vi "Display Module Info.vi"(8 "error IO":errorcluster, 11 "Array":refnum<class "Module.lvclass">[](array[class])) -> (0 "error out":errorcluster, 3 "Array 2":refnum<class "Module.lvclass">[](array[class]))   [LabVIEW 2021, in "Module.lvclass"]
uses:
  Module.lvclass
  Module.lvclass/Module.ctl
  <vilib>/printing/OpenHTMLReport.llb/Open HTML Report in Browser (Refnum).vi
  <vilib>/Utility/NIReport.llb/NI_report.lvclass
  <vilib>/Utility/NIReport.llb/NI_ReportGenerationCore.lvlib
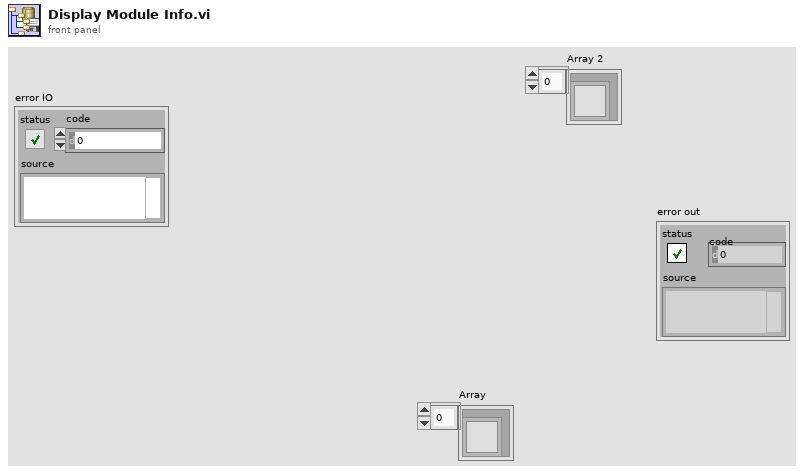
[diagram p1: front panel]
types:
  T1 = enum16{"Standard Report", "HTML", "Word", "Excel"}
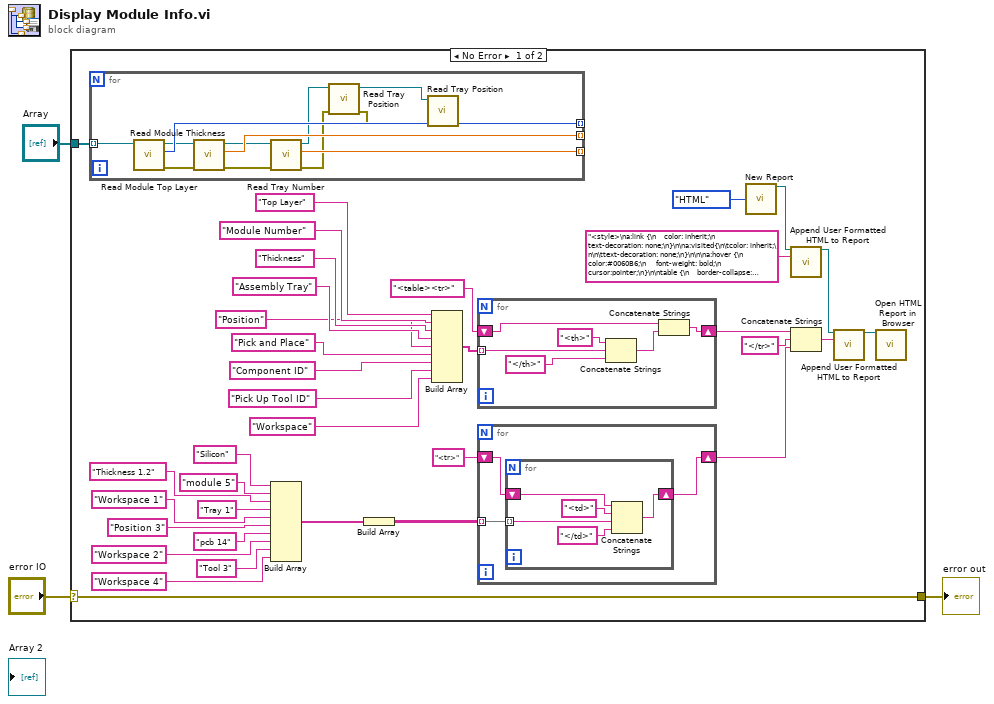
[diagram p0: block diagram]
diagram:
  n1 = case shown="No Error" "error IO" {
    selector: "error IO" -> [w38 w65]
    tunnel: [w38 w65] -> w3
    tunnel: "Array" -> [w4 _]
    frame No Error {
      n2 = for {
        tunnel: w4 -> [w50] mode=indexing
        tunnel: [w49] -> _ mode=indexing
        tunnel: [w46] -> _ mode=indexing
        tunnel: [w43] -> _ mode=indexing
        n3 = call "Read Module Top Layer.vi"("Module in"=w50) -> ("error out"=w48:errorcluster, "Module Top Layer"=w49:enum16{"Baseplate", "Kapton", "Sensor", "PCB"}, "Module out"=w47:refnum<class "Module.lvclass">)  [unwired: 8 in]
        n4 = call "Read Module Thickness.vi"("error in (no error)"=w48, "Module in"=w47) -> ("error out"=w44:errorcluster, "Module Thickness"=w46:dbl, "Module out"=w45:refnum<class "Module.lvclass">)  [unwired: 7 in]
        n5 = call "Read Tray Number.vi"("error in (no error)"=w44, "Module in"=w45) -> ("error out"=w41:errorcluster, "Tray Number"=w43:dbl, "Module out"=w42:refnum<class "Module.lvclass">)  [unwired: 7 in]
        n6 = call "Read Tray Position.vi"("error in (no error)"=w41, "Module in"=w42) -> ("error out"=w39:errorcluster, "Module out"=w40:refnum<class "Module.lvclass">)  [unwired: 7 in, 1 out]
        n7 = call "Read Tray Position.vi"("error in (no error)"=w39, "Module in"=w40) -> ()  [unwired: 7 in, 3 out]
      }
      n8 = Build Array("Silicon" ("element"), "module 5" ("element"), "Thickness 1.2" ("element"), "Tray 1" ("element"), "Workspace 1" ("element"), "Position 3" ("element"), "pcb 14" ("element"), "Workspace 2" ("element"), "Tool 3" ("element"), "Workspace 4" ("element")) -> (w31:string[])
      n9 = Build Array(w31) -> (w8:string[][])
      n10 = Build Array("Top Layer", "Module Number", "Thickness", "Assembly Tray" ("element"), "Position" ("element"), "Pick and Place" ("element"), "Component ID" ("element"), "Pick Up Tool ID" ("element"), "Workspace" ("element")) -> (w15:string[])
      n11 = for {
        tunnel: w15 -> [w62] mode=indexing
        shift-right: [w59] -> w13
        shift-left: "<table><tr>" ("HTML text") -> [w61]
        n12 = Concatenate Strings("<th>", w62, "</th>") -> (w60:string)
        n13 = Concatenate Strings(w61, w60) -> (w59:string)
      }
      n14 = for {
        tunnel: w8 -> [w52] mode=indexing
        shift-right: [w51] -> w6
        shift-left: "<tr>" -> [w53]
        n15 = for {
          shift-right: [w56] -> w51
          shift-left: w53 -> [w58]
          tunnel: w52 -> [w55] mode=indexing
          n16 = Concatenate Strings(w58, "<td>", w55, "</td>") -> (w56:string)
        }
      }
      n17 = call <vilib>:"New Report.vi"("report type"=T1."HTML") -> ("report out"=w10:refnum<class "NI_report.lvclass">)  [unwired: 13 in, 1 out]
      n18 = call-dynamic "Append User Formatted HTML to Report.vi"("report in"=w10, "HTML text"="<style>\na:link {\n    color: inherit;\n    text-decoration: none;\n}\n\na:visited{\n\tcolor: inherit;\n\n\ttext-decoration: none;\n}\n\n\na:hover {\n     color:#0060B6;\n     font-weight: bold;\n     cursor:pointer;\n}\n\ntable {\n    border-collapse: collapse;\n    width: 100%;\n\tmargin-top: 30px;    \n\tmargin-bottom: 30px;\n}\n\nth, td {\n    padding: 10px;\n    spacing: 5px;\n    text-align: left;\n    border-bottom: 1px solid #ddd;\n}\n\ntr:hover{background-color:#f5f5f5}\n\nnav {\n\tfloat: left;\n\twidth: 150px;\n\tborder: 1px solid;\n}\n\nsection {\n    margin-left: 175px;\n\n}\n</style>" ("text")) -> ("report out"=w9:refnum<class "NI_report.lvclass">)  [unwired: 12 in, 1 out]
      n19 = Concatenate Strings(w13, "</tr>" ("string"), w6) -> (w11:string)
      n20 = call-dynamic "Append User Formatted HTML to Report.vi"("report in"=w9, "HTML text"=w11) -> ("report out"=w5:refnum<class "NI_report.lvclass">)  [unwired: 12 in, 1 out]
      n21 = call-poly <vilib>:"Open HTML Report in Browser.vi"("report in"=w5) -> ()  [unwired: 12 in, 3 out]
    }
    frame Error {
    }
  }
  "error out" <- w3
